vi "(SubVI) DAC(write) Rate Options_YCC.vi"(4 "DAC to write waiting time per point (ms)\nrange from 5ms to 0.167 ms":dbl=5.0) -> (0 "In Range?\n5ms to0.167ms":bool, 1 "In Range waiting time to write (ms)":dbl)   [LabVIEW 2014]
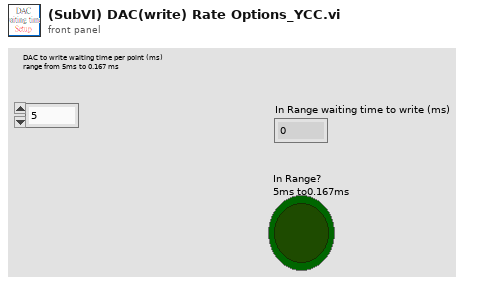
[diagram p1: front panel]
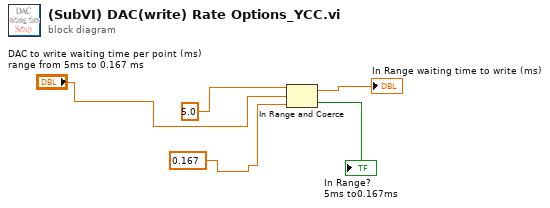
[diagram p0: block diagram]
diagram:
  n1 = In Range and Coerce(upper limit=5.0 ("y"), x="DAC to write waiting time per point (ms)\nrange from 5ms to 0.167 ms", lower limit=0.167 ("y")) -> (coerced(x)=→"In Range waiting time to write (ms)":dbl, In Range?=→"In Range?\n5ms to0.167ms":bool)
